vi "Send SetPower Message.vi"(8 "error in (no error)":errorcluster, 10 "PowerData":T1, 11 "Execute":refnum<class "Execute.lvclass">) -> (0 "error out":errorcluster, 3 "Execute 2":refnum<class "Execute.lvclass">)   [LabVIEW 2018, in "QMH_Class.lvlib" / "TestManager.lvlib" / "SetPower Message.lvclass"]
uses:
  SetPower Message.lvclass
  Execute_class/Execute.lvclass
  E:/0 File/GITSync/DynoToolPlus/0 LabviewCode/0 Support/Message Queue_Class/Class/Message_class/InterfaceMessage/Interface Message.lvclass
  SetPower Message.lvclass/SetPower Message.ctl
  Execute_class/Execute.lvclass/Execute.ctl
  InterfaceMessage/Interface Message.lvclass
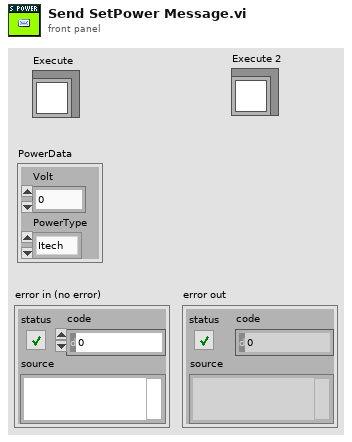
[diagram p1: front panel]
types:
  T1 = cluster{"Volt":dbl, "PowerType":enum16{"Itech", "Keysight"}}
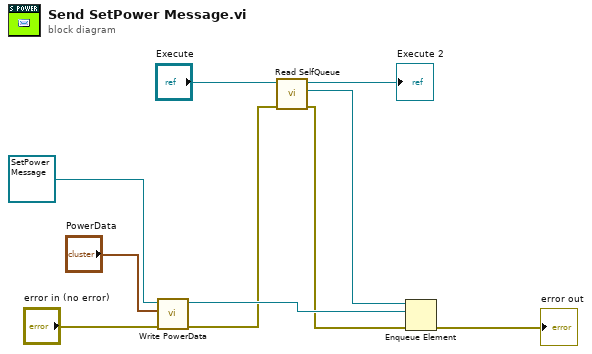
[diagram p0: block diagram]
diagram:
  n1 = call "Write PowerData.vi"("error in (no error)"="error in (no error)", "PowerData"="PowerData", "SetPower Message"=refnum<class "SetPower Message.lvclass"> refnum ("QMH_Class.lvlib:TestManager.lvlib:SetPower Message.lvclass")) -> ("error out"=w3:errorcluster, "SetPower Message"=w9:refnum<class "SetPower Message.lvclass">)  [unwired: 7 in]
  n2 = call "Read SelfQueue.vi"("error in (no error)"=w3, "Execute"="Execute") -> ("error out"=w2:errorcluster, "SelfQueue"=w1:refnum<queue>, "Execute"=→"Execute 2":refnum<class "Execute.lvclass">)  [unwired: 7 in]
  n3 = Enqueue Element(queue=w1, element=w9, error in (no error)=w2) -> (error out=→"error out":errorcluster)  [unwired: 1 in, 2 out]
